vi "Solve for Dz.vi"(4 "end":dbl=1e-05 format="%#g", 5 "start":dbl format="%#g", 6 "n":i32=6, 7 "mu":dbl=1.836922107566826e-05, 8 "error in":errorcluster, 9 "P":dbl=10113.0, 10 "T":dbl=293.15, 11 "Z1":dbl=3.2561526610201098e-09) -> (0 "error out":errorcluster, 3 "dz":dbl)   [LabVIEW 2015]
doc: "This VI solves the equation Z(n=1)-n*e*Cc(D)/(3*pi*mu*D)=0 to determine the diameter of multiply charged particles."
uses:
  DMA Data.ctl
  <vilib>/gmath/zero.llb/Find All Zeros of f(x) (VI).vi
  <vilib>/gmath/NI_Gmath.lvlib
  DMA.lvclass
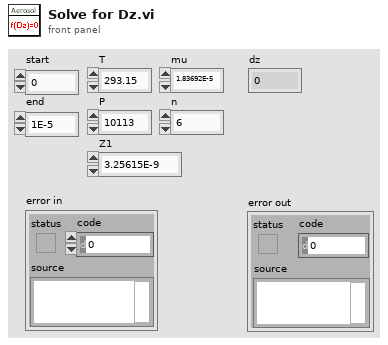
[diagram p1: front panel]
types:
  T1 = typedef "DMA.lvclass/DMA Data.ctl" = cluster{"T":dbl, "P":dbl, "n":i32, "mu":dbl, "Z1":dbl}
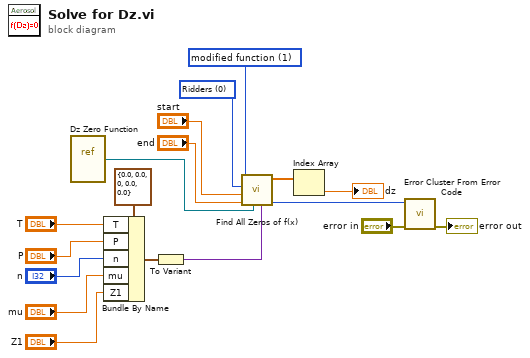
[diagram p0: block diagram]
diagram:
  w3 = u16 0 items=["Ridders", "Newton Raphson"] ("algorithm")
  w4 = u16 1 items=["fixed function", "modified function"] ("step type")
  n1 = vi-ref "Dz Zero Function.vi"() -> (w18:refnum<vi>)
  n2 = Bundle By Name(cluster=T1 {"T"=0.0, "P"=0.0, "n"=0, "mu"=0.0, "Z1"=0.0}, "T"="T", "P"="P", "n"="n", "mu"="mu", "Z1"="Z1") -> (w10:T1)
  n3 = To Variant(anything=w10) -> (Variant=w9:variant)
  n4 = call-poly <vilib>:"Find All Zeros of f(x).vi"("data"=w9, "f(x)"=w18, "end"="end", "start"="start", "algorithm"=w3, "step type"=w4) -> ("error"=w8:i32, "Zeros"=w2:dbl[])  [unwired: 2 in, 2 out]
  n5 = Index Array(array=w2) -> (element=→"dz":dbl)  [unwired: 1 in]
  n6 = call <vilib>:"Error Cluster From Error Code.vi"("error in (no error)"="error in", "error code (0)"=w8) -> ("error out"=→"error out":errorcluster)  [unwired: 7 in]
